vi "example_chatmodel_unit_test_1.vi"() -> ()   [LabVIEW 2020]
uses:
  src/models/abstract_llm_chatcompletion/abstract_llm_chatcompletion.lvclass
  src/models/message_text/message_text.lvclass
  D:/petwork/labview-llm-libraries/src/models/abstract_message_base/abstract_message_base.lvclass
  src/models/llm_openai_chatmodels/llm_openai_chatmodels.lvclass
  D:/petwork/labview-llm-libraries/src/models/abstract_llm_base/abstract_llm_base.lvclass
  src/models/llm_azureopenai_chatmodels/llm_azureopenai_chatmodels.lvclass
  src/models/llm_anthropic_chatmodels/llm_anthropic_chatmodels.lvclass
  src/models/llm_ollama_chatmodels/llm_ollama_chatmodels.lvclass
  src/models/message_text/create_text_message.vi
  src/models/llm_openai_chatmodels/Instantiate_llm_openai.vi
  src/models/llm_azureopenai_chatmodels/Instantiate_llm_azureopenai.vi
  src/models/llm_anthropic_chatmodels/Instantiate_llm_anthropic.vi
  src/models/llm_ollama_chatmodels/Instantiate_llm_ollama.vi
  src/models/message_text/get_text_message_value.vi
  src/models/abstract_llm_base/abstract_llm_base.lvclass
panel:
  in  "Provider Selector":T1(tab)
  in  "model_name":string(combo)="gpt-4o-mini"
  out "openai_key":string
  in  "temperature":dbl=1.0
  in  "Messages":cluster{"role":string, "text":string}[](array[cluster])=[{"role"="system", "text"="Act as a math teacher and guide the student in solving the problem. You should not solve the problem. Always answer in single line."}, {"role"="user", "text"="What is x in the equation 2x + 3 = 5  ?"}]
  out "error out":errorcluster
  # "1. Ensure you assign the OpenAI Key to environmental variables so it is away from the code and easy to use the examples in future.\n\n2. Use the \"Set_ENv_Var.vi\" from examples/utils folder to set the key \"labview_llm_openai_key\"."
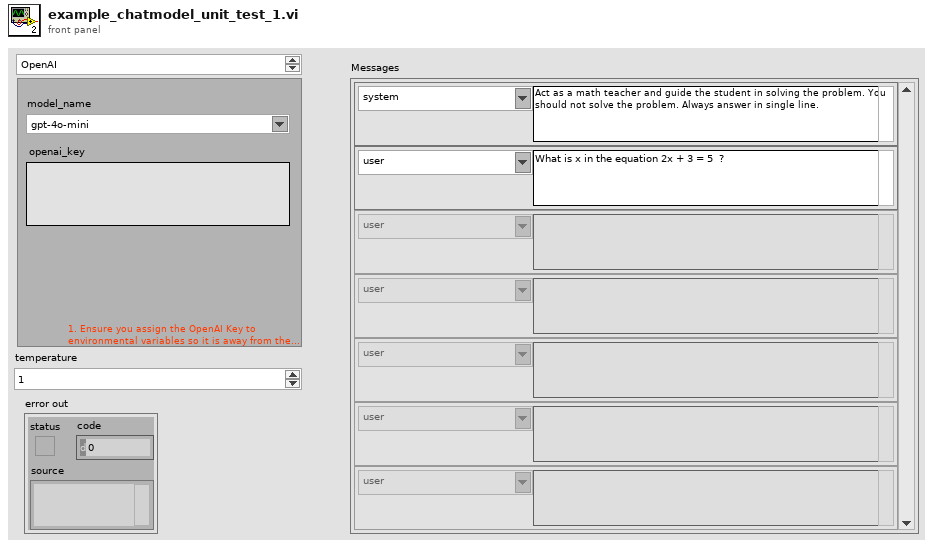
[diagram p1: front panel]
types:
  T1 = enum32{"OpenAI", "Azure OpenAI", "Anthropic", "Ollama"}
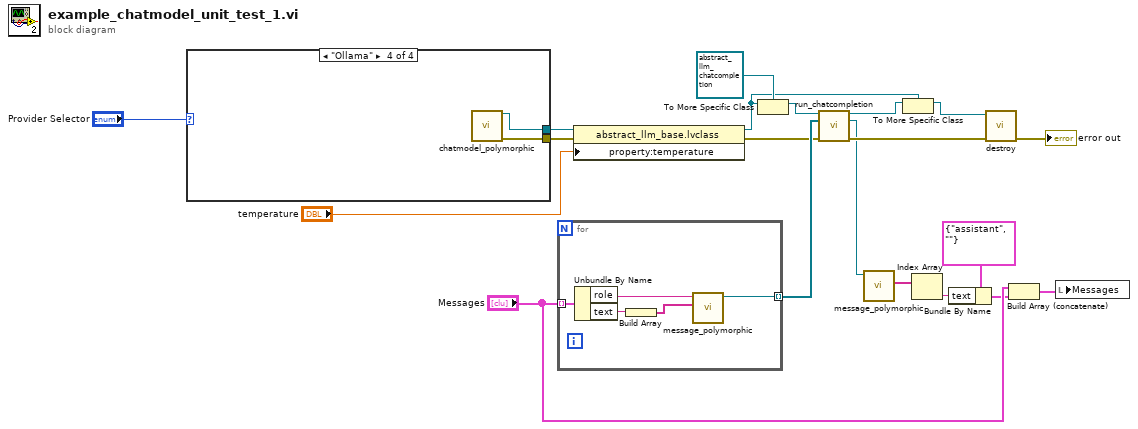
[diagram p0: block diagram]
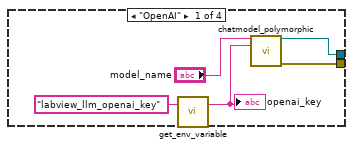
[diagram p2: hidden frame]
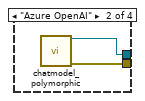
[diagram p3: hidden frame]
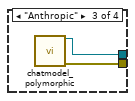
[diagram p4: hidden frame]
diagram:
  n1 = case shown="\"Ollama\"" "Provider Selector" {
    tunnel: [w24 w27 w29 w30] -> w8
    tunnel: [w23 w26 w28 w31] -> w6
    frame "OpenAI" {
      n2 = call "get_env_variable.vi"("Environment Variable Name"="labview_llm_openai_key") -> ("Value"=w21:string)  [unwired: 1 in, 1 out]
      "openai_key" <- w21
      n3 = call-poly "chatmodel_polymorphic.vi"("model_name"="model_name", "openai_key"=w21) -> ("llm_openai out"=w23:refnum<class "llm_openai_chatmodels.lvclass">, "error out"=w24:errorcluster)  [unwired: 12 in]
    }
    frame "Azure OpenAI" {
      n4 = call-poly "chatmodel_polymorphic.vi"() -> ("llm_azureopenai_chatmodels out"=w26:refnum<class "llm_azureopenai_chatmodels.lvclass">, "error out"=w27:errorcluster)  [unwired: 14 in]
    }
    frame "Anthropic" {
      n5 = call-poly "chatmodel_polymorphic.vi"() -> ("llm_anthropic_chatmodels out"=w28:refnum<class "llm_anthropic_chatmodels.lvclass">, "error out"=w29:errorcluster)  [unwired: 14 in]
    }
    frame "Ollama" {
      n6 = call-poly "chatmodel_polymorphic.vi"() -> ("llm_openai out"=w31:refnum<class "llm_ollama_chatmodels.lvclass">, "error out"=w30:errorcluster)  [unwired: 14 in]
    }
  }
  n7 = for {
    tunnel: "Messages" -> [w36] mode=indexing
    tunnel: [w32] -> w18 mode=indexing
    n8 = Unbundle By Name(w36) -> ("role"=w34:string, "text"=w35:string)
    n9 = Build Array(w35) -> (w33:string[])
    n10 = call-poly "message_polymorphic.vi"("content"=w33, "role"=w34) -> ("message_text out"=w32:refnum<class "message_text.lvclass">)  [unwired: 8 in, 1 out]
  }
  n11 = property class="abstract_llm_base.lvclass"(reference=w6, error in=w8, "property:temperature"="temperature") -> (reference out=w2:refnum<class "abstract_llm_base.lvclass">, error out=w15:errorcluster)
  n12 = To More Specific Class(target class=refnum<class "abstract_llm_chatcompletion.lvclass"> refnum ("chatcompletion_llm_interface in"), reference=w2) -> (specific class reference=w4:refnum<class "abstract_llm_chatcompletion.lvclass">)  [unwired: 1 in, 1 out]
  n13 = call-dynamic "run_chatcompletion.vi"("chatcompletion_llm_interface in"=w4, "Messages"=w18, "error in (no error)"=w15) -> ("chatcompletion_llm_interface out"=w3:refnum<class "abstract_llm_chatcompletion.lvclass">, "Response"=w10:refnum<class "abstract_message_base.lvclass">, "error out"=w20:errorcluster)  [unwired: 10 in]
  n14 = call-poly "message_polymorphic.vi"("abstract_message_base.lvclass"=w10) -> ("content"=w9:string[])  [unwired: 8 in, 2 out]
  n15 = To More Specific Class(target class=w2, reference=w3) -> (specific class reference=w1:refnum<class "abstract_llm_base.lvclass">)  [unwired: 1 in, 1 out]
  n16 = Index Array(array=w9) -> (element=w12:string)  [unwired: 1 in]
  n17 = Bundle By Name(cluster=cluster{"role":string, "text":string} {"role"="assistant", "text"=""} ("message"), "text"=w12) -> (w11:cluster{"role":string, "text":string})
  n18 = call-dynamic "destroy.vi"("error in (no error)"=w20, "abstract_llm_base in"=w1) -> ("error out"=→"error out":errorcluster)  [unwired: 8 in, 1 out]
  n19 = Build Array (concatenate)("Messages", w11) -> (w16:cluster{"role":string, "text":string}[])
  n20 = local write "Messages"(w16) -> ()
